vi "ALL.vi"   [LabVIEW 2016, in "LVtoITX.lvclass"]
uses:
  LVtoITX.lvclass
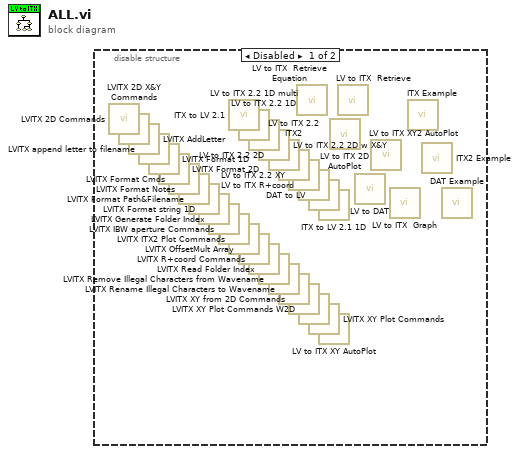
[diagram p0: block diagram]
diagram:
  n1 = disable-structure shown="Disabled" {
    frame Disabled {
      n2 = call "LVITX 2D Commands.vi"() -> ()  [unwired: 15 in, 1 out]
      n3 = call "LVITX 2D X&Y Commands.vi"() -> ()  [unwired: 10 in, 2 out]
      n4 = call "LVITX AddLetter.vi"() -> ()  [unwired: 1 in, 1 out]
      n5 = call "LVITX append letter to filename.vi"() -> ()  [unwired: 1 in, 1 out]
      n6 = call "LVITX Format 1D.vi"() -> ()  [unwired: 2 in, 1 out]
      n7 = call "LVITX Format 2D.vi"() -> ()  [unwired: 2 in, 1 out]
      n8 = call "LVITX Format Cmds.vi"() -> ()  [unwired: 1 in, 1 out]
      n9 = call "LVITX Format Notes.vi"() -> ()  [unwired: 1 in, 1 out]
      n10 = call "LVITX Format Path&Filename.vi"() -> ()  [unwired: 2 in, 2 out]
      n11 = call "LVITX Format string 1D.vi"() -> ()  [unwired: 2 in, 1 out]
      n12 = call "LVITX Generate Folder Index.vi"() -> ()  [unwired: 12 in]
      n13 = call "LVITX IBW aperture Commands.vi"() -> ()  [unwired: 4 in, 1 out]
      n14 = call "ITX to LV 2.1.vi"() -> ()  [unwired: 2 in, 4 out]
      n15 = call "LVITX ITX2 Plot Commands.vi"() -> ()  [unwired: 6 in, 1 out]
      n16 = call "LV to ITX 2.2 1D multi.vi"() -> ()  [unwired: 12 in]
      n17 = call "LVITX OffsetMult Array.vi"() -> ()  [unwired: 3 in, 1 out]
      n18 = call "LV to ITX 2.2 1D.vi"() -> ()  [unwired: 12 in]
      n19 = call "LVITX R+coord Commands.vi"() -> ()  [unwired: 15 in, 1 out]
      n20 = call "LV to ITX 2.2 2D w X&Y.vi"() -> ()  [unwired: 11 in, 1 out]
      n21 = call "LVITX Read Folder Index.vi"() -> ()  [unwired: 11 in, 1 out]
      n22 = call "LV to ITX 2.2 2D.vi"() -> ()  [unwired: 12 in]
      n23 = call "LVITX Remove Illegal Characters from Wavename.vi"() -> ()  [unwired: 1 in, 1 out]
      n24 = call "LV to ITX 2.2 ITX2.vi"() -> ()  [unwired: 11 in, 1 out]
      n25 = call "LVITX Rename Illegal Characters to Wavename.vi"() -> ()  [unwired: 1 in, 1 out]
      n26 = call "LV to ITX 2.2 XY.vi"() -> ()  [unwired: 11 in, 1 out]
      n27 = call "LVITX XY from 2D Commands.vi"() -> ()  [unwired: 2 in, 1 out]
      n28 = call "LV to ITX  Retrieve Equation.vi"() -> ()  [unwired: 11 in, 5 out]
      n29 = call "LV to ITX R+coord.vi"() -> ()  [unwired: 12 in]
      n30 = call "LVITX XY Plot Commands W2D.vi"() -> ()  [unwired: 5 in, 1 out]
      n31 = call "DAT to LV.vi"() -> ()  [unwired: 9 in, 3 out]
      n32 = call "LVITX XY Plot Commands.vi"() -> ()  [unwired: 6 in, 1 out]
      n33 = call "ITX to LV 2.1 1D.vi"() -> ()  [unwired: 7 in, 5 out]
      n34 = call "LV to ITX XY AutoPlot.vi"() -> ()  [unwired: 15 in, 1 out]
      n35 = call "LV to ITX 2D AutoPlot.vi"() -> ()  [unwired: 15 in, 1 out]
      n36 = call "LV to ITX  Retrieve.vi"() -> ()  [unwired: 11 in, 5 out]
      n37 = call "LV to DAT.vi"() -> ()  [unwired: 11 in, 1 out]
      n38 = call "LV to ITX XY2 AutoPlot.vi"() -> ()  [unwired: 15 in, 1 out]
      n39 = call "LV to ITX  Graph.vi"() -> ()  [unwired: 12 in]
      n40 = call "ITX Example.vi"() -> ()  [unwired: 12 in]
      n41 = call "ITX2 Example.vi"() -> ()  [unwired: 12 in]
      n42 = call "DAT Example.vi"() -> ()  [unwired: 12 in]
    }
    frame Enabled {
    }
  }
